vi "REPORT_GEAR_delete_ID_column.vi"(11 "REPORT_GEAR_all_info":T1) -> (3 "REPORT_GEAR_all_info_ID_deleted":T1)   [LabVIEW 2019]
uses:
  typedef/REPORT_GEAR_all_info.ctl
  typedef/REPORT_GEAR_header_data_display.ctl
  typedef/REPORT_GEAR_statuses.ctl
panel:
  # "GEAR INFO SUMMARY"
  # "GEAR INFO SUMMARY"
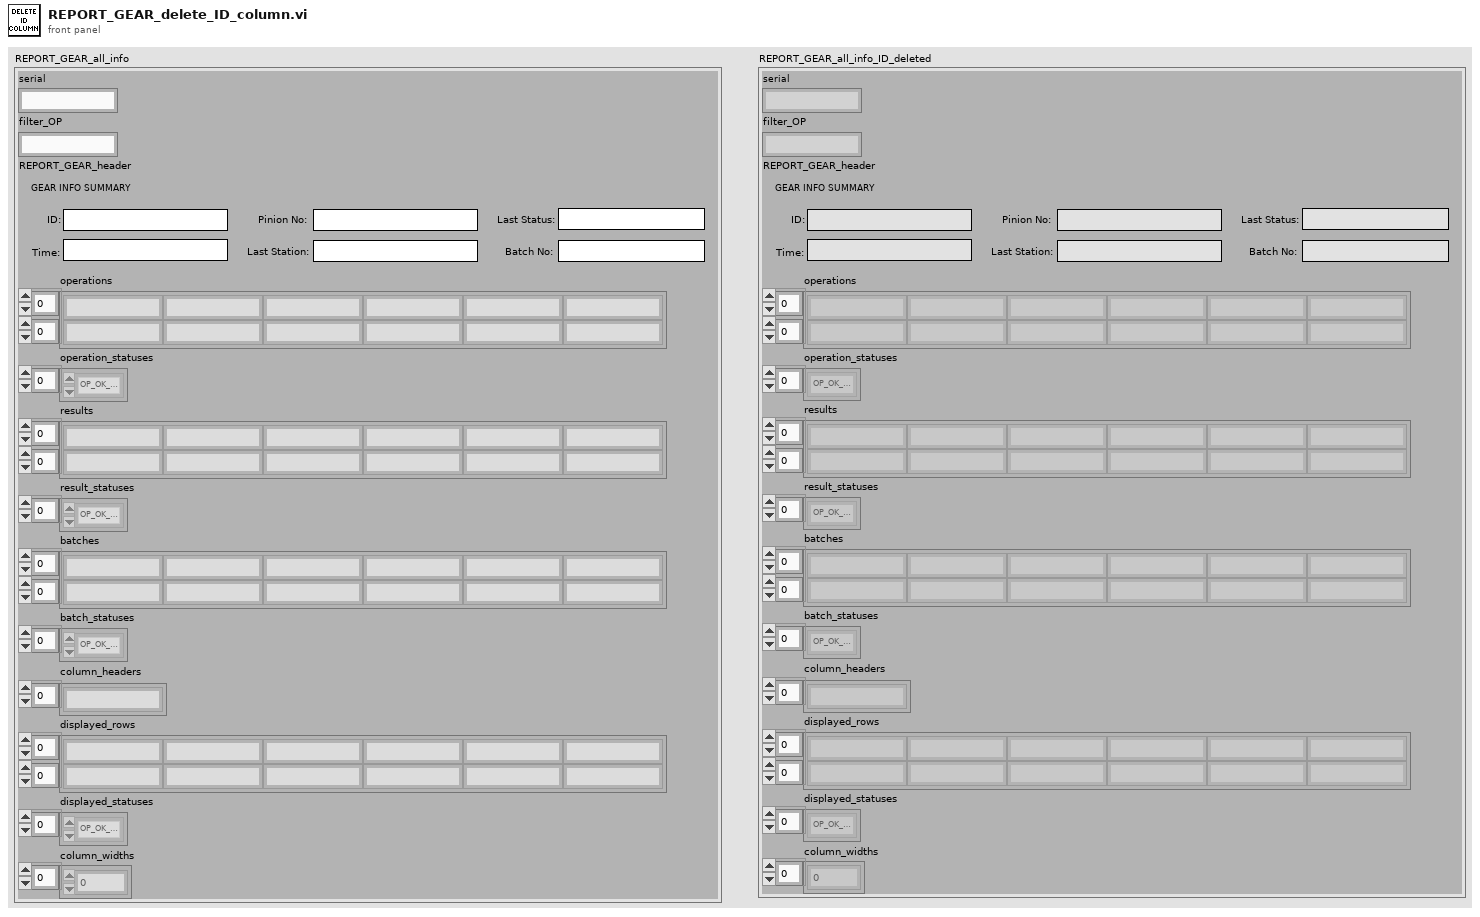
[diagram p1: front panel]
types:
  T1 = typedef "REPORT_GEAR_all_info.ctl" = cluster{"serial":string, "filter_OP":string, "REPORT_GEAR_header":T2, "operations":string[][], "operation_statuses":T3[], "results":string[][], "result_statuses":T3[], "batches":string[][], "batch_statuses":T3[], "column_headers":string[], "displayed_rows":string[][], "displayed_statuses":T3[], "column_widths":i16[]}
  T2 = typedef "REPORT_GEAR_header_data_display.ctl" = cluster{"ID":string, "creation_time":string, "last_station":string, "last_status":string, "pinion_serial":string, "batch_code":string}
  T3 = typedef "REPORT_GEAR_statuses.ctl" = enum16{"OP_OK_hide", "OP_OK_show", "OP_NOK_hide", "OP_NOK_show", "OP_interrupted_hide", "OP_interrupted_show", "OP_in_operation_hide", "OP_in_operation_show", "OP_unexpected_hide", "OP_unexpected_show", "RE_REAL_OK", "RE_REAL_NOK", "RE_STRING", "RE_sub_header", "RE_no_data", "RE_unexpected", "BA_sub_header", "BA_data", "BA_no_data"}
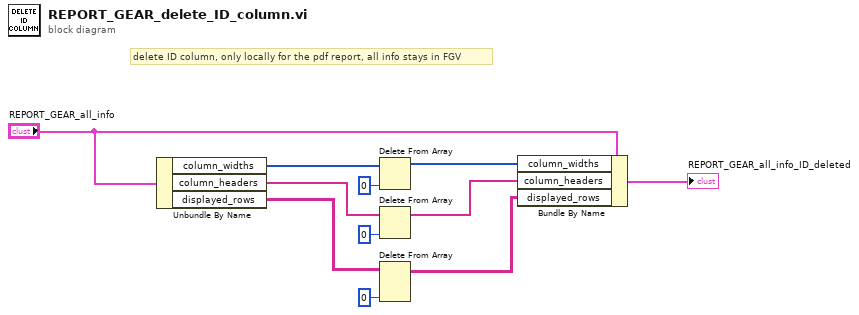
[diagram p0: block diagram]
diagram:
  # "delete ID column, only locally for the pdf report, all info stays in FGV"
  n1 = Unbundle By Name("REPORT_GEAR_all_info") -> ("column_widths"=w11:i16[], "column_headers"=w10:string[], "displayed_rows"=w9:string[][])
  n2 = Delete From Array(array=w11, index=0) -> (array with subset deleted=w3:i16[])  [unwired: 1 in, 1 out]
  n3 = Delete From Array(array=w10, index=0) -> (array with subset deleted=w2:string[])  [unwired: 1 in, 1 out]
  n4 = Delete From Array(array=w9, index (col)=0 ("disabled index (col)")) -> (array with subset deleted=w1:string[][])  [unwired: 2 in, 1 out]
  n5 = Bundle By Name(cluster="REPORT_GEAR_all_info", "column_widths"=w3, "column_headers"=w2, "displayed_rows"=w1) -> (→"REPORT_GEAR_all_info_ID_deleted":T1)
